vi "readAnalogInputChannel.vi"(0 "Controller in":refnum<class "_Controller.lvclass">, 2 "ai_channel (def=1)":u8=1, 5 "error in (no error)":errorcluster) -> (14 "Controller out":refnum<class "_Controller.lvclass">, 16 "value (V)":dbl, 19 "error out":errorcluster)   [LabVIEW 2013, in "classes.lvlib" / "_Controller.lvclass"]
doc: "Acquire a single analog voltage value at the specified analog input (AI) channel\n\nProduced By:\n\n<B>Kod Integrations, LLC</B>\n4835 Marianne Drive\nMount Airy, MD 21771\nhttp://www.kodintegrations.com\nemail: info@kodintegrations.com\nphone: (240) 687-1288"
uses:
  _Controller.lvclass
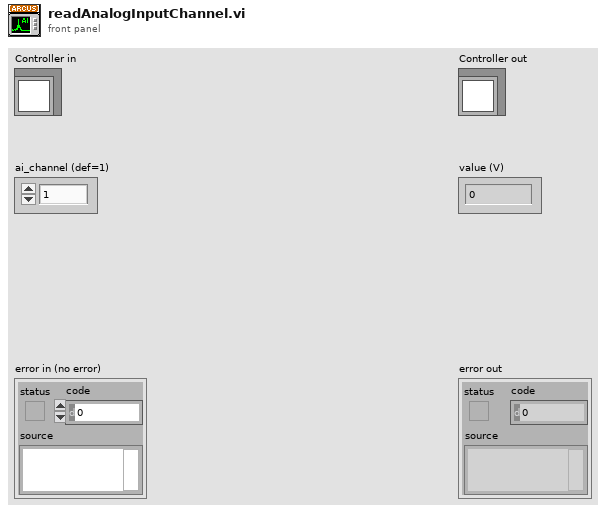
[diagram p1: front panel]
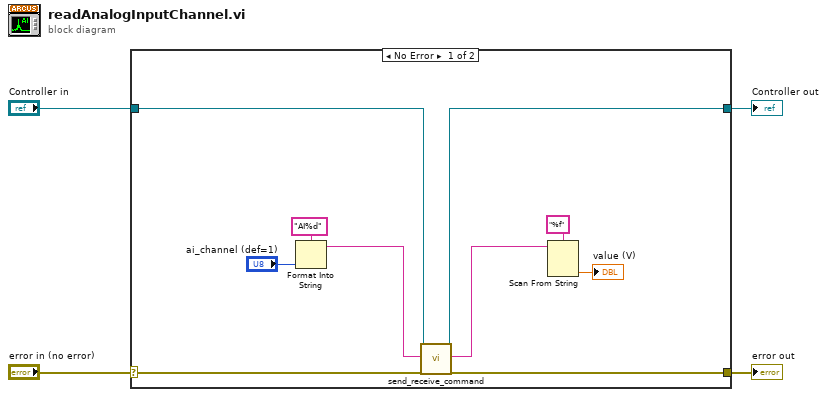
[diagram p0: block diagram]
diagram:
  n1 = case shown="No Error" "error in (no error)" {
    selector: "error in (no error)" -> [w14 w16]
    tunnel: [w13 w16] -> w3
    tunnel: [w11 w15] -> w1
    tunnel: "Controller in" -> [w12 w15]
    frame No Error {
      n2 = Format Into String(format string="AI%d", "ai_channel (def=1)") -> (resulting string=w8:string)  [unwired: 2 in, 1 out]
      n3 = call "send_receive_command.vi"("reference (in)"=w12, "ASCII Command (in)"=w8, "error in (no error)"=w14) -> ("reference (out)"=w11:refnum<class "_Controller.lvclass">, "response (out)"=w6:string, "error out"=w13:errorcluster)  [unwired: 12 in, 2 out]
      n4 = Scan From String(format string="%f", input string=w6) -> (output 1=→"value (V)":dbl)  [unwired: 3 in, 3 out]
    }
    frame Error {
    }
  }
  "error out" <- w3
  "Controller out" <- w1
